vi "VSS_GoTo_Circ.vi"(6 "Npoint":i32, 9 "y 3":dbl=0.5, 10 "SetPoint":dbl[](array[numeric])=[100.0, 100.0, 0.0], 11 "Position":dbl[](array[numeric])=[208.6539306640625, -200.4281768798828, 3.141592653589793]) -> (3 "Output Vel":dbl[](array[numeric])=[0.0, 0.0, 0.8321627905647668])   [LabVIEW 2018]
uses:
  <vilib>/Analysis/_algsub.llb/Real Vector Norm.vi
  <vilib>/Analysis/coordinate.llb/Wrap Angle (scalar).vi
  <vilib>/Analysis/NI_AAL_Angle.lvlib
  <vilib>/Analysis/NI_AALPro.lvlib
panel:
  in  "Beta":dbl=0.17
  in  "Dmin":dbl=250.0
  in  "fc angular":dbl=80.0
  out "Angular":dbl(graph)=0.8321627905647668
  out "Tangent":dbl(graph)
  in  "fc tangent":dbl=0.85
  out "NaN":bool
  in  "y 2":dbl=20.0 format="%#_13g"
  in  "y":dbl=0.6 format="%#_13g"
  in  "Limits tangent":cluster{"output high":dbl, "output low":dbl}={"output high"=1.2, "output low"=-1.2}
  in  "PID gains tangent":T1={"proportional gain (Kc)"=0.0044, "integral time (Ti, min)"=0.0, "derivative time (Td, min)"=-0.085}
  in  "Limits ang":cluster{"output high":dbl, "output low":dbl}={"output high"=1.0, "output low"=-1.0}
  in  "PID gains ang":T1={"proportional gain (Kc)"=0.5, "integral time (Ti, min)"=0.0, "derivative time (Td, min)"=-0.08}
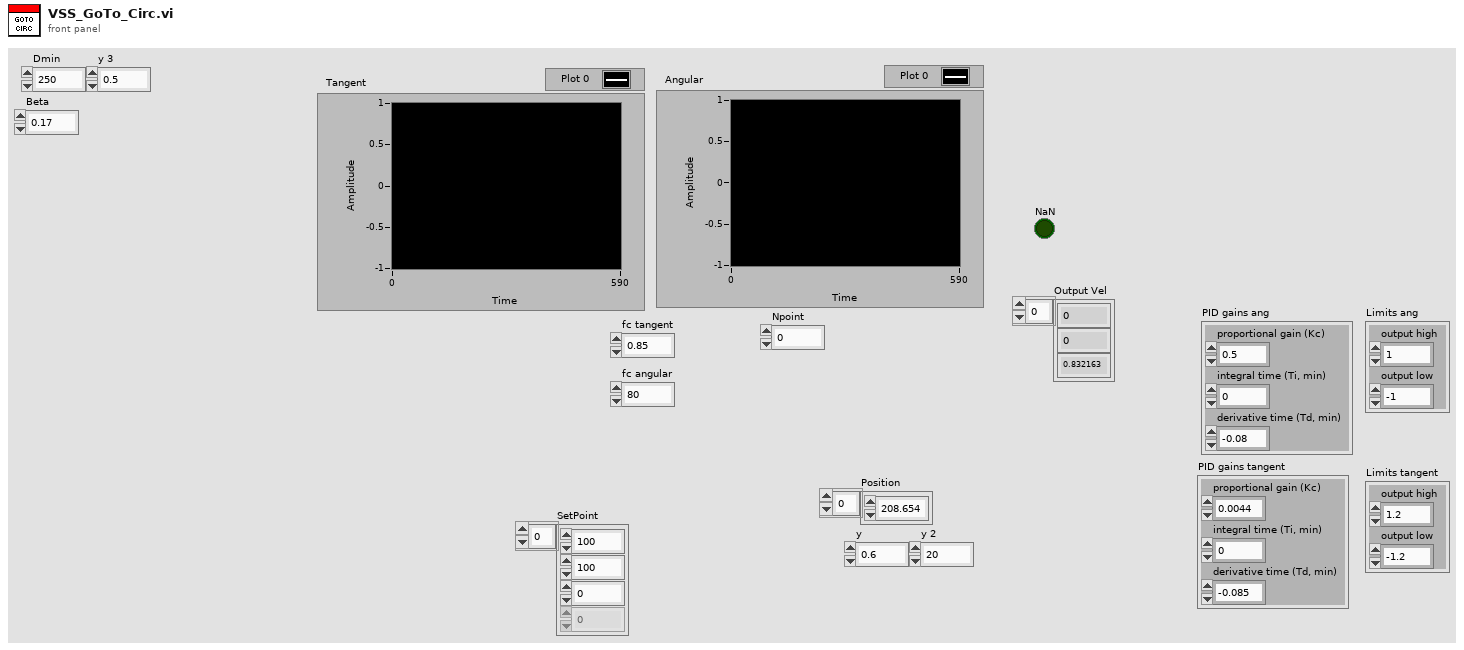
[diagram p1: front panel]
types:
  T1 = cluster{"proportional gain (Kc)":dbl, "integral time (Ti, min)":dbl, "derivative time (Td, min)":dbl}
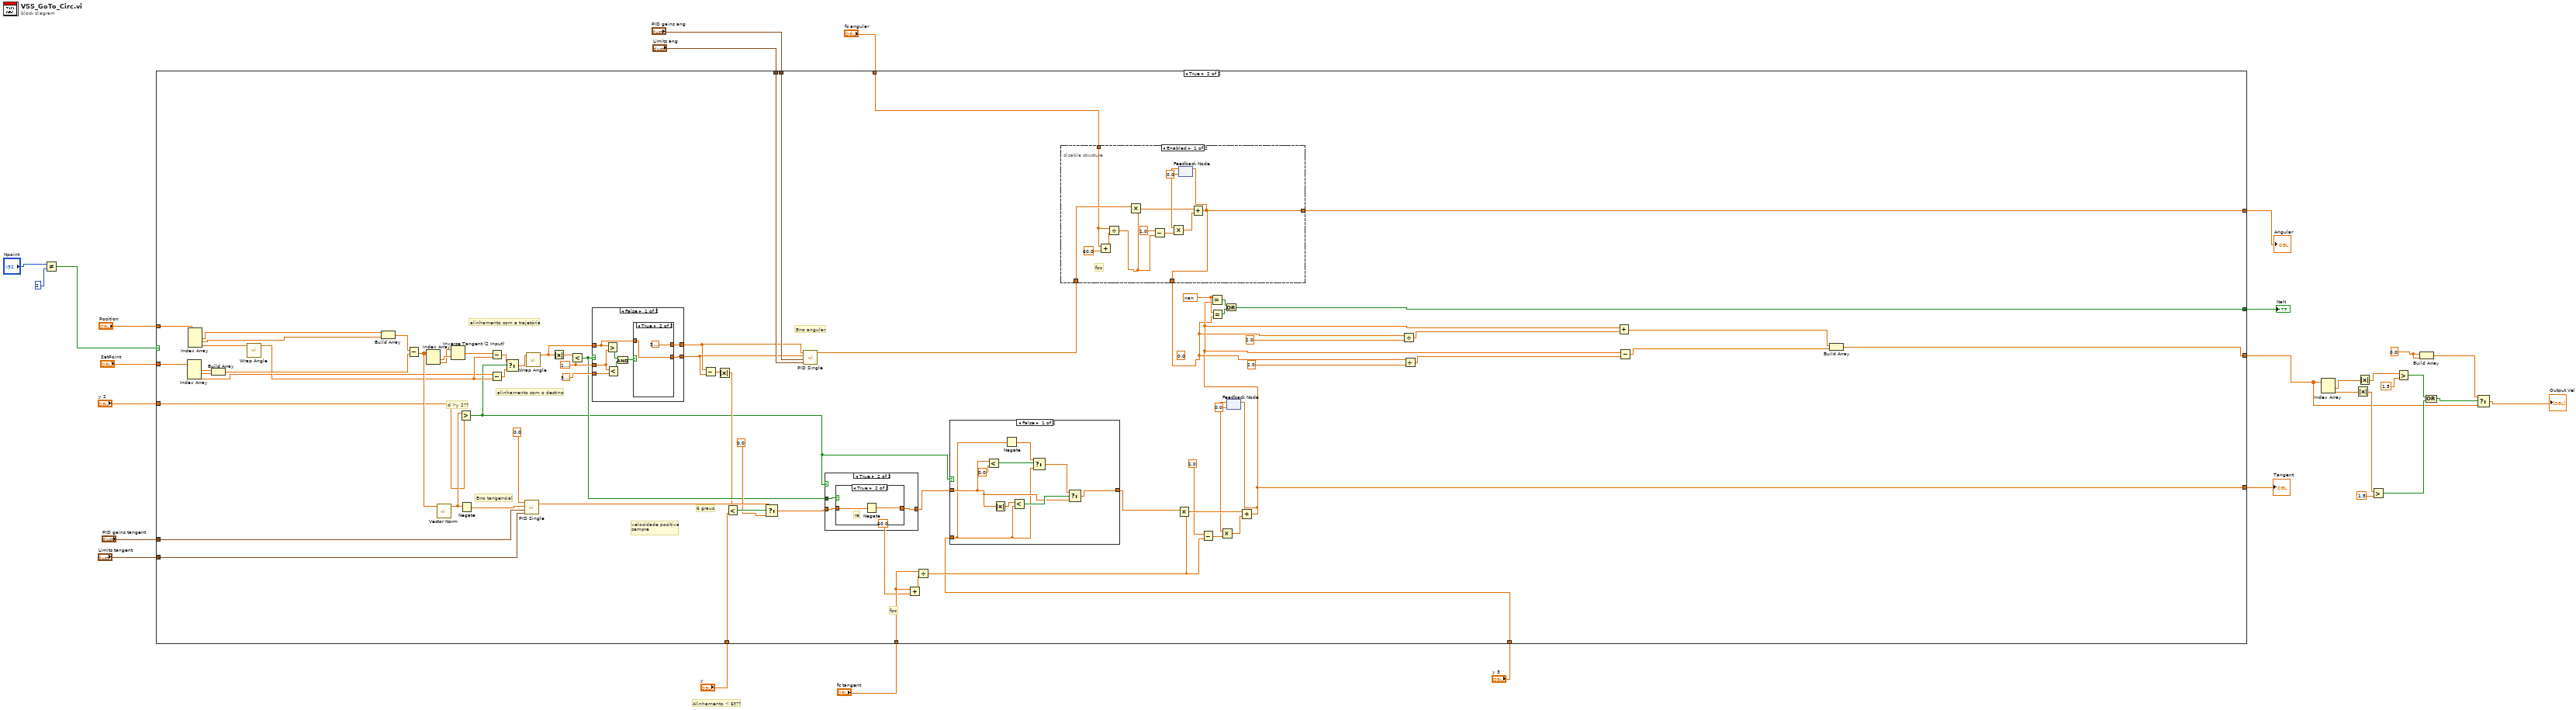
[diagram p0: block diagram]
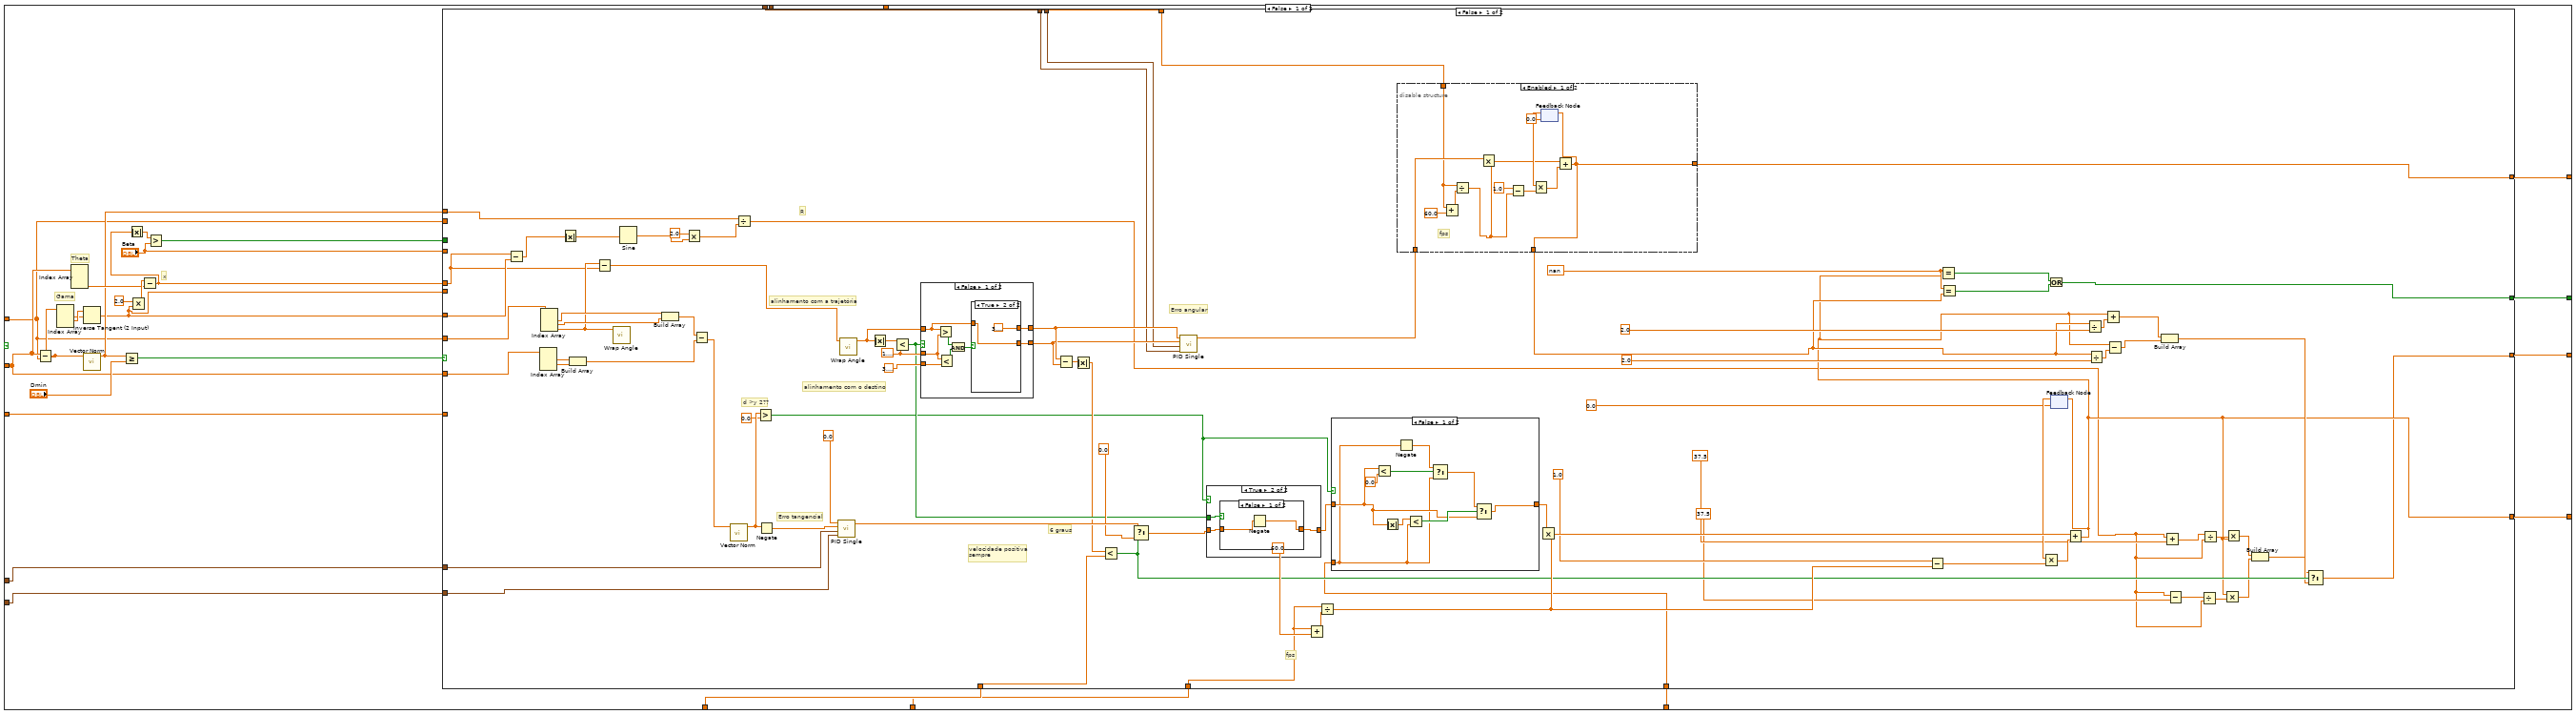
[diagram p2: hidden frame]
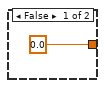
[diagram p5: hidden frame]
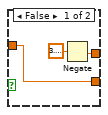
[diagram p7: hidden frame]
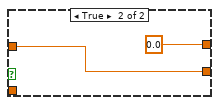
[diagram p8: hidden frame]
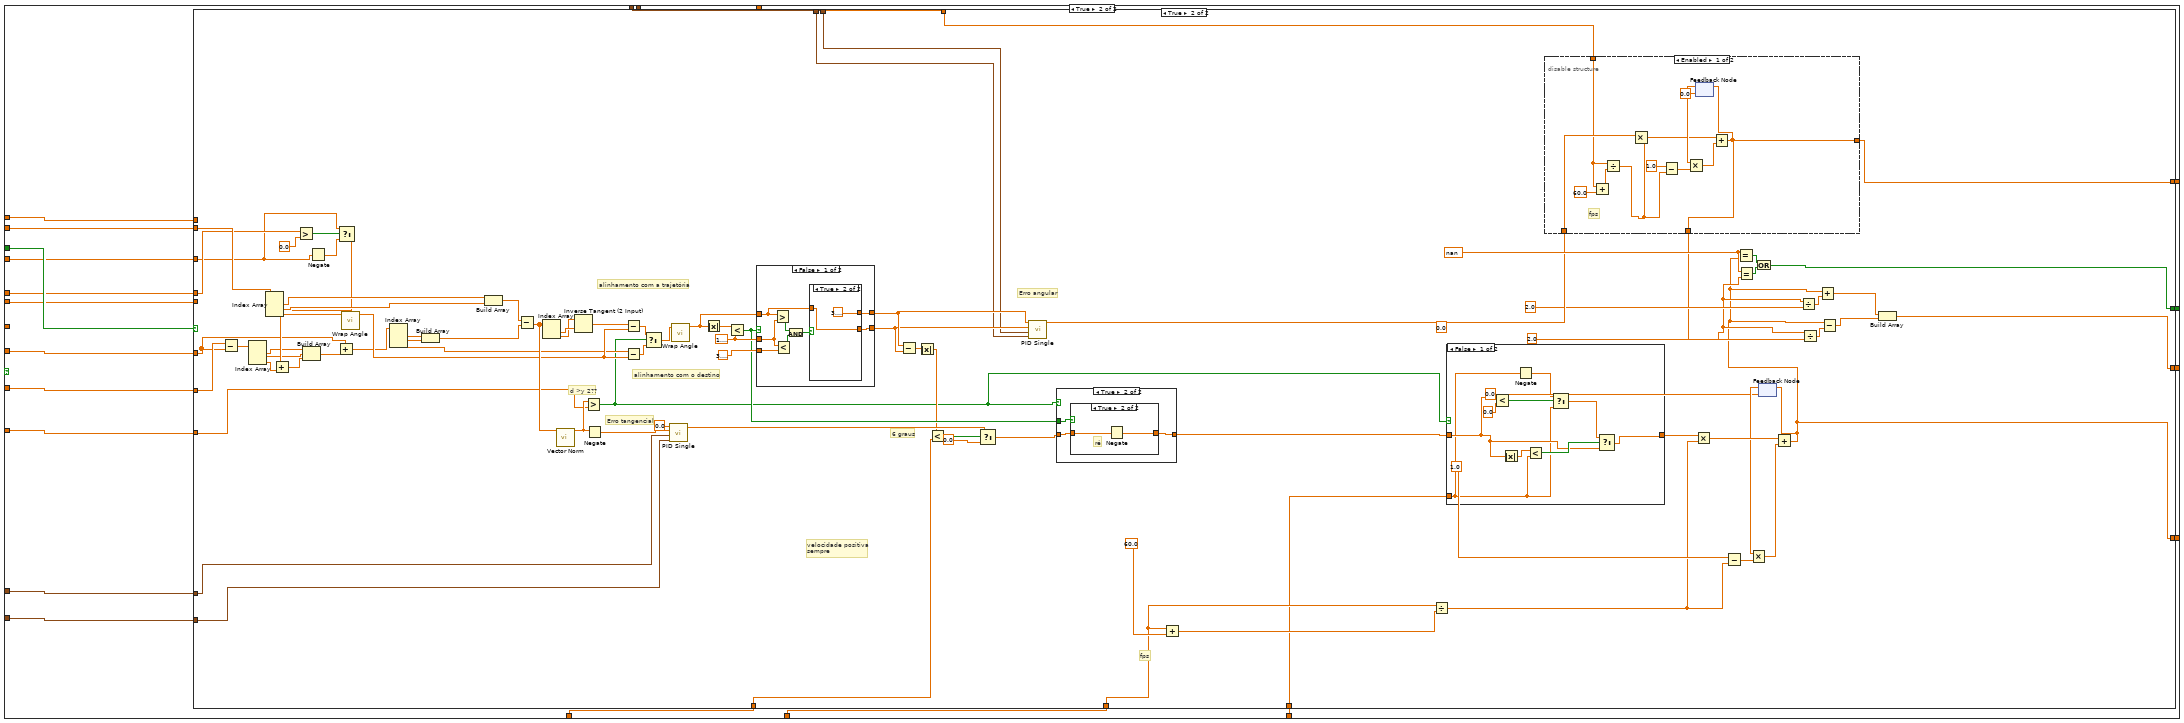
[diagram p9: hidden frame]
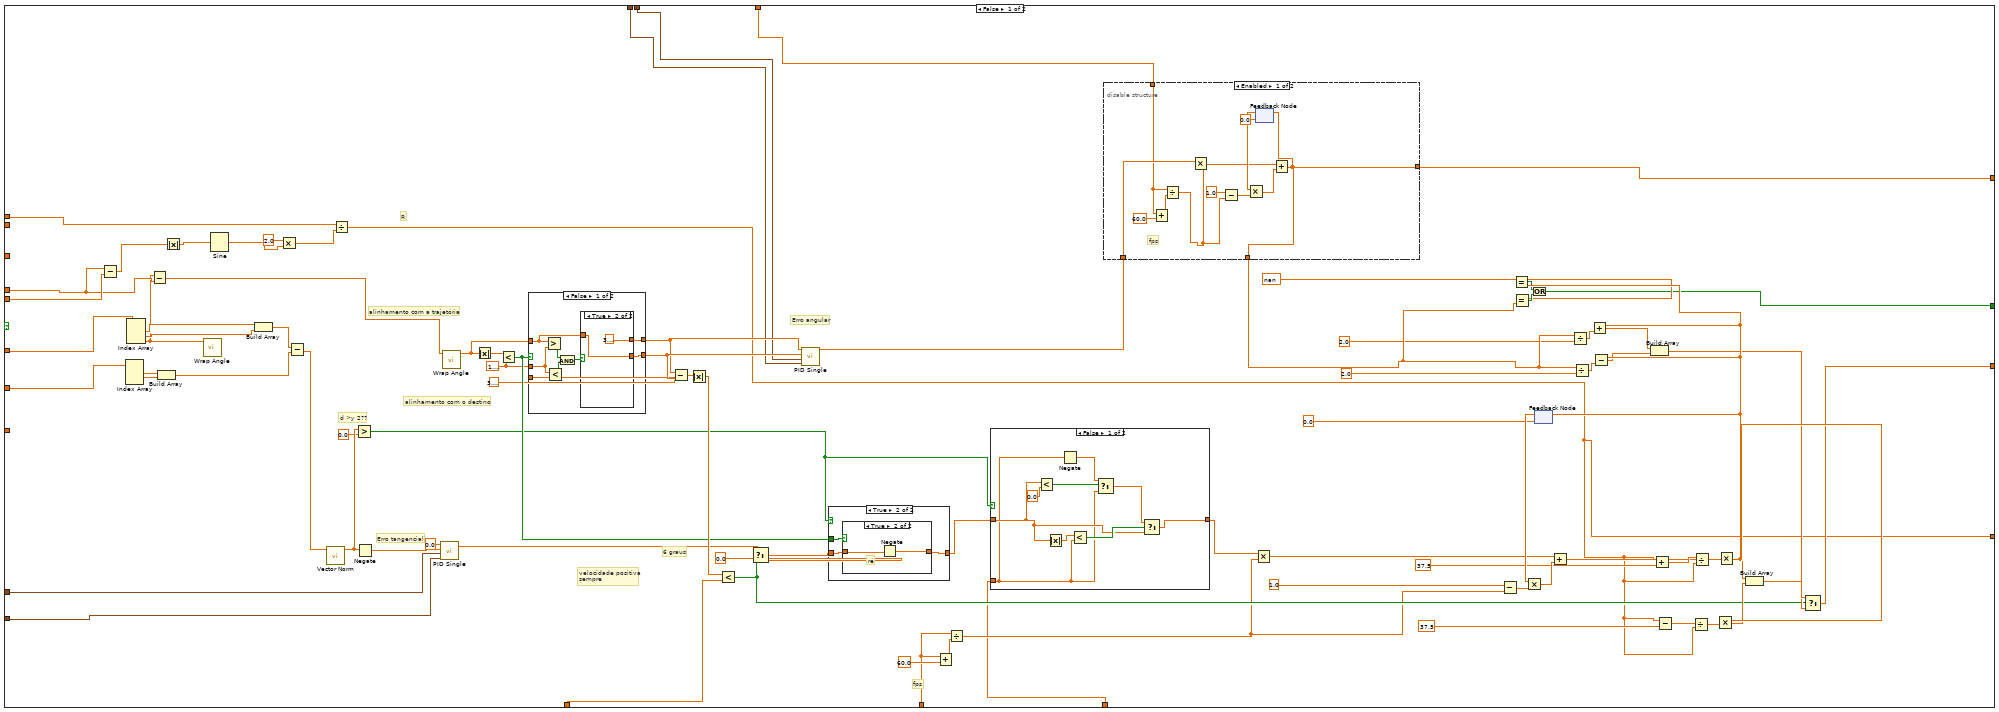
[diagram p10: hidden frame]
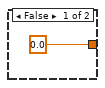
[diagram p13: hidden frame]
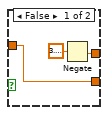
[diagram p15: hidden frame]
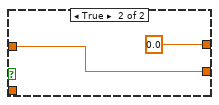
[diagram p16: hidden frame]
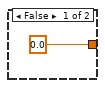
[diagram p19: hidden frame]
diagram:
  w3 = 0.0 ("element")
  # "Alinhamento < 6º??"
  n1 = Not Equal?(x="Npoint", y=2) -> (x != y?=w15:bool)
  n2 = case shown="True" w15 {
    tunnel: "Position" -> [w36 w533]
    tunnel: "PID gains tangent" -> [w50 w528]
    tunnel: "Limits tangent" -> [w51 w527]
    tunnel: "y" -> [w53 w526]
    tunnel: "SetPoint" -> [w48 w520]
    tunnel: "PID gains ang" -> [w46 w516]
    tunnel: "Limits ang" -> [w47 w515]
    tunnel: "y 2" -> [w49 w495]
    tunnel: [w43 w490] -> w22
    tunnel: "fc tangent" -> [w52 w482]
    tunnel: [w41 w470] -> w20
    tunnel: [w42 w468] -> w4
    tunnel: [w44 w478] -> w19
    tunnel: "fc angular" -> [w45 w477]
    tunnel: "y 3" -> [w31 w464]
    frame False {
      # "x"
      # "Theta"
      # "Gama"
      n3 = Subtract(x=w48, y=w36) -> (x-y=w57:dbl[])
      n4 = Index Array(array=w57) -> (element #1=w33:dbl, element #2=w34:dbl)  [unwired: 3 in, 1 out]
      n5 = Index Array(array=w48) -> (element #3=w54:dbl)  [unwired: 3 in, 2 out]
      n6 = Inverse Tangent (2 Input)(1:w33, 2:w34) -> (0:w32:dbl)
      n7 = call-poly <vilib>:"Vector Norm.vi"("Input Vector"=w57) -> ("norm"=w40:dbl)  [unwired: 9 in, 1 out]
      n8 = Greater Or Equal?(x=w40, y="Dmin") -> (x >= y?=w58:bool)
      n9 = Multiply(x=2.0, y=w32) -> (x*y=w55:dbl)
      n10 = Subtract(x=w55, y=w54) -> (x-y=w38:dbl)
      n11 = Absolute Value(x=w38) -> (abs(x)=w37:dbl)
      n12 = Greater?(x=w37, y="Beta") -> (0:w39:bool)
      n13 = case shown="False" w58 {
        tunnel: w38 -> [w64 w205]
        tunnel: w53 -> [w106 w199]
        tunnel: w52 -> [w105 w198]
        tunnel: w51 -> [w104 w200]
        tunnel: w50 -> [w103 w201]
        tunnel: w49 -> [_ w202]
        tunnel: w36 -> [w102 w204]
        tunnel: w48 -> [w101 w203]
        tunnel: w47 -> [w100 w196]
        tunnel: w46 -> [w99 w197]
        tunnel: w45 -> [w98 w189]
        tunnel: [w97 w190] -> w44
        tunnel: [w96 w195] -> w43
        tunnel: [w71 w194] -> w42
        tunnel: [w75 w193] -> w41
        tunnel: w40 -> [w92 w206]
        tunnel: w39 -> [_ w207]
        tunnel: w36 -> [_ w192]
        tunnel: "Beta" -> [_ w191]
        tunnel: w32 -> [w69 _]
        tunnel: w32 -> [_ w188]
        tunnel: w31 -> [w60 w187]
        frame False {
          w119 = nan
          w131 = 1.5707963267948966
          # "R"
          # "d >y 2??"
          # "fps"
          # "alinhamento com o destino"
          # "alinhamento com a trajetória"
          # "velocidade positiva\nsempre"
          # "Erro tangencial"
          # "Erro angular"
          # "6 graus"
          n14 = Subtract(x=w64, y=w69) -> (x-y=w66:dbl)
          n15 = Index Array(array=w101) -> (element #1=w135:dbl, element #2=w134:dbl)  [unwired: 3 in, 1 out]
          n16 = Index Array(array=w102) -> (element #1=w137:dbl, element #2=w136:dbl, element #3=w65:dbl)  [unwired: 3 in]
          n17 = Absolute Value(x=w66) -> (abs(x)=w67:dbl)
          n18 = Build Array(w135, w134) -> (w133:dbl[])
          n19 = Subtract(x=w65, y=w64) -> (x-y=w68:dbl)
          n20 = call-poly <vilib>:"Wrap Angle.vi"("angle in"=w65) -> ()  [unwired: 9 in, 2 out]
          n21 = Sine(x=w67) -> (sin(x)=w94:dbl)
          n22 = Build Array(w137, w136) -> (w141:dbl[])
          n23 = Multiply(x=2.0, y=w94) -> (x*y=w93:dbl)
          n24 = Subtract(x=w141, y=w133) -> (x-y=w122:dbl[])
          n25 = call-poly <vilib>:"Vector Norm.vi"("Input Vector"=w122) -> ("norm"=w121:dbl)  [unwired: 9 in, 1 out]
          n26 = Divide(x=w92, y=w93) -> (x/y=w72:dbl)
          n27 = Greater?(x=w121, y=0.0) -> (0:w61:bool)
          n28 = Negate(x=w121) -> (-x=w126:dbl)
          n29 = call "PID Single.vi"("Limits"=w104, "PID gains in"=w103, "Variable"=w126, "Setpoint"=0.0) -> ("Out"=w139:dbl)  [unwired: 7 in]
          n30 = call-poly <vilib>:"Wrap Angle.vi"("angle in"=w68) -> ("angle out"=w129:dbl)  [unwired: 9 in, 1 out]
          n31 = Absolute Value(x=w129) -> (abs(x)=w132:dbl)
          n32 = Less?(x=w132, y=w131) -> (x < y?=w127:bool)
          n33 = case shown="False" w127 {
            tunnel: w129 -> [w172 w186]
            tunnel: [w173 w186] -> w124
            tunnel: w131 -> [w179 _]
            tunnel: 3.141592653589793 -> [w178 _]
            tunnel: [w174 0.0 ("Variable")] -> w125
            frame False {
              n34 = Greater?(x=w172, y=w179) -> (0:w176:bool)
              n35 = Less?(x=w179, y=w178) -> (x < y?=w177:bool)
              n36 = And(x=w176, y=w177) -> (x .and. y?=w175:bool)
              n37 = case shown="True" w175 {
                tunnel: [w182 3.141592653589793] -> w174
                tunnel: [w180 w183] -> w173
                tunnel: w172 -> [w180 w183]
                frame False {
                  n38 = Negate(x=3.141592653589793) -> (-x=w182:dbl)
                }
                frame True {
                }
              }
            }
            frame True {
            }
          }
          n39 = Subtract(x=w125, y=w124) -> (x-y=w123:dbl)
          n40 = Absolute Value(x=w123) -> (abs(x)=w120:dbl)
          n41 = Less?(x=w120, y=w106) -> (x < y?=w87:bool)
          n42 = Select(t=w139, s=w87, f=0.0) -> (s? t:f=w128:dbl)
          n43 = call "PID Single.vi"("Limits"=w100, "PID gains in"=w99, "Variable"=w124, "Setpoint"=w125) -> ("Out"=w107:dbl)  [unwired: 7 in]
          n44 = case shown="True" w61 {
            tunnel: w128 -> [_ w168]
            tunnel: w127 -> [_ w167]
            tunnel: [0.0 ("f") w166] -> w62
            frame False {
            }
            frame True {
              n45 = case shown="False" w167 {
                tunnel: w168 -> [w170 w171]
                tunnel: [w169 w171] -> w166
                frame False {
                  n46 = Negate(x=w170) -> (-x=w169:dbl)
                }
                frame True {
                  # "ré"
                }
              }
            }
          }
          n47 = Add(x=w105, y=60.0) -> (x+y=w108:dbl)
          n48 = Divide(x=w105, y=w108) -> (x/y=w110:dbl)
          n49 = case shown="False" w61 {
            tunnel: w62 -> [w144 w151]
            tunnel: w60 -> [w143 _]
            tunnel: [w142 w151] -> w63
            frame False {
              n50 = Less?(x=w144, y=0.0) -> (x < y?=w147:bool)
              n51 = Absolute Value(x=w144) -> (abs(x)=w150:dbl)
              n52 = Negate(x=w143) -> (-x=w146:dbl)
              n53 = Less?(x=w150, y=w143) -> (x < y?=w149:bool)
              n54 = Select(t=w146, s=w147, f=w143) -> (s? t:f=w145:dbl)
              n55 = Select(t=w145, s=w149, f=w144) -> (s? t:f=w142:dbl)
            }
            frame True {
            }
          }
          n56 = disable-structure shown="Enabled" {
            disable-tunnel: [w153 w164] -> w86
            disable-tunnel: w107 -> [w154 w164]
            disable-tunnel: [w153 _] -> w97
            disable-tunnel: w98 -> [w152 _]
            frame Enabled {
              # "fps"
              n57 = Add(x=w152, y=60.0) -> (x+y=w157:dbl)
              n58 = Divide(x=w152, y=w157) -> (x/y=w155:dbl)
              n59 = Multiply(x=w154, y=w155) -> (x*y=w158:dbl)
              n60 = Subtract(x=1.0, y=w155) -> (x-y=w160:dbl)
              n61 = feedback #1(0.0) -> (w161:dbl)
              n62 = Multiply(x=w161, y=w160) -> (x*y=w162:dbl)
              n63 = Add(x=w158, y=w162) -> (x+y=w153:dbl)
              n64 = feedback-in #1(w153) -> ()
            }
            frame Disabled {
            }
          }
          n65 = Multiply(x=w63, y=w110) -> (x*y=w116:dbl)
          n66 = Subtract(x=1.0, y=w110) -> (x-y=w114:dbl)
          n67 = Equal?(x=w119, y=w86) -> (x = y?=w118:bool)
          n68 = feedback #2(0.0) -> (w113:dbl)
          n69 = Multiply(x=w113, y=w114) -> (x*y=w112:dbl)
          n70 = Add(x=w116, y=w112) -> (x+y=w75:dbl)
          n71 = Equal?(x=w119, y=w75) -> (x = y?=w117:bool)
          n72 = Or(x=w117, y=w118) -> (x .or. y?=w96:bool)
          n73 = feedback-in #2(w75) -> ()
          n74 = Divide(x=w86, y=2.0) -> (x/y=w88:dbl)
          n75 = Divide(x=w86, y=2.0) -> (x/y=w91:dbl)
          n76 = Add(x=w75, y=w88) -> (x+y=w85:dbl)
          n77 = Subtract(x=w75, y=w91) -> (x-y=w84:dbl)
          n78 = Build Array(w85, w84) -> (w83:dbl[])
          n79 = Add(x=w72, y=37.5) -> (x+y=w73:dbl)
          n80 = Subtract(x=w72, y=37.5) -> (x-y=w74:dbl)
          n81 = Divide(x=w74, y=w72) -> (x/y=w80:dbl)
          n82 = Divide(x=w73, y=w72) -> (x/y=w76:dbl)
          n83 = Multiply(x=w75, y=w80) -> (x*y=w79:dbl)
          n84 = Multiply(x=w76, y=w75) -> (x*y=w78:dbl)
          n85 = Build Array(w78, w79) -> (w77:dbl[])
          n86 = Select(t=w77, s=w87, f=w83) -> (s? t:f=w71:dbl[])
        }
        frame True {
          n87 = case shown="True" w207 {
            tunnel: w206 -> [w232 _]
            tunnel: w205 -> [w213 w361]
            tunnel: w204 -> [w231 w350]
            tunnel: w203 -> [w230 w357]
            tunnel: w202 -> [_ w364]
            tunnel: w201 -> [w229 w365]
            tunnel: w200 -> [w228 w366]
            tunnel: w199 -> [w227 w347]
            tunnel: w198 -> [w226 w346]
            tunnel: w197 -> [w224 w340]
            tunnel: w196 -> [w223 w341]
            tunnel: [w222 w345] -> w195
            tunnel: [w221 w343] -> w194
            tunnel: [w220 w342] -> w193
            tunnel: w192 -> [_ w363]
            tunnel: w191 -> [_ w359]
            tunnel: [w219 w344] -> w190
            tunnel: w189 -> [w225 w339]
            tunnel: w188 -> [w217 _]
            tunnel: w187 -> [w209 w335]
            frame False {
              w241 = nan
              w245 = 1.5707963267948966
              # "R"
              # "d >y 2??"
              # "fps"
              # "alinhamento com o destino"
              # "alinhamento com a trajetória"
              # "velocidade positiva\nsempre"
              # "Erro tangencial"
              # "Erro angular"
              # "6 graus"
              n88 = Subtract(x=w213, y=w217) -> (x-y=w215:dbl)
              n89 = Index Array(array=w230) -> (element #1=w250:dbl, element #2=w251:dbl)  [unwired: 3 in, 1 out]
              n90 = Index Array(array=w231) -> (element #1=w248:dbl, element #2=w249:dbl, element #3=w212:dbl)  [unwired: 3 in]
              n91 = Subtract(x=w212, y=w213) -> (x-y=w216:dbl)
              n92 = Build Array(w250, w251) -> (w252:dbl[])
              n93 = Absolute Value(x=w215) -> (abs(x)=w214:dbl)
              n94 = call-poly <vilib>:"Wrap Angle.vi"("angle in"=w212) -> ()  [unwired: 9 in, 2 out]
              n95 = Sine(x=w214) -> (sin(x)=w273:dbl)
              n96 = Build Array(w248, w249) -> (w246:dbl[])
              n97 = Multiply(x=2.0, y=w273) -> (x*y=w274:dbl)
              n98 = Subtract(x=w246, y=w252) -> (x-y=w261:dbl[])
              n99 = call-poly <vilib>:"Vector Norm.vi"("Input Vector"=w261) -> ("norm"=w262:dbl)  [unwired: 9 in, 1 out]
              n100 = Divide(x=w232, y=w274) -> (x/y=w220:dbl)
              n101 = Greater?(x=w262, y=0.0) -> (0:w211:bool)
              n102 = Negate(x=w262) -> (-x=w257:dbl)
              n103 = call "PID Single.vi"("Limits"=w228, "PID gains in"=w229, "Variable"=w257, "Setpoint"=0.0) -> ("Out"=w247:dbl)  [unwired: 7 in]
              n104 = call-poly <vilib>:"Wrap Angle.vi"("angle in"=w216) -> ("angle out"=w254:dbl)  [unwired: 9 in, 1 out]
              n105 = Absolute Value(x=w254) -> (abs(x)=w253:dbl)
              n106 = Less?(x=w253, y=w245) -> (x < y?=w256:bool)
              n107 = case shown="False" w256 {
                tunnel: w254 -> [w320 w334]
                tunnel: [w321 w334] -> w259
                tunnel: w245 -> [w327 _]
                tunnel: 3.141592653589793 -> [w326 _]
                tunnel: [w322 0.0 ("Variable")] -> w258
                frame False {
                  n108 = Greater?(x=w320, y=w327) -> (0:w324:bool)
                  n109 = Less?(x=w327, y=w326) -> (x < y?=w325:bool)
                  n110 = And(x=w324, y=w325) -> (x .and. y?=w323:bool)
                  n111 = case shown="True" w323 {
                    tunnel: [w330 3.141592653589793] -> w322
                    tunnel: [w328 w331] -> w321
                    tunnel: w320 -> [w328 w331]
                    frame False {
                      n112 = Negate(x=3.141592653589793) -> (-x=w330:dbl)
                    }
                    frame True {
                    }
                  }
                }
                frame True {
                }
              }
              n113 = Subtract(x=w258, y=w259) -> (x-y=w260:dbl)
              n114 = Absolute Value(x=w260) -> (abs(x)=w263:dbl)
              n115 = Less?(x=w263, y=w227) -> (x < y?=w277:bool)
              n116 = Select(t=w247, s=w277, f=0.0) -> (s? t:f=w255:dbl)
              n117 = call "PID Single.vi"("Limits"=w223, "PID gains in"=w224, "Variable"=w259, "Setpoint"=w258) -> ("Out"=w272:dbl)  [unwired: 7 in]
              n118 = case shown="True" w211 {
                tunnel: w255 -> [_ w316]
                tunnel: w256 -> [_ w315]
                tunnel: [0.0 ("f") w314] -> w208
                frame False {
                }
                frame True {
                  n119 = case shown="True" w315 {
                    tunnel: w316 -> [w317 w319]
                    tunnel: [w317 w318] -> w314
                    frame False {
                    }
                    frame True {
                      # "ré"
                      n120 = Negate(x=w319) -> (-x=w318:dbl)
                    }
                  }
                }
              }
              n121 = Add(x=w226, y=60.0) -> (x+y=w271:dbl)
              n122 = Divide(x=w226, y=w271) -> (x/y=w270:dbl)
              n123 = case shown="False" w211 {
                tunnel: w208 -> [w292 w299]
                tunnel: w209 -> [w291 _]
                tunnel: [w290 w299] -> w210
                frame False {
                  n124 = Less?(x=w292, y=0.0) -> (x < y?=w295:bool)
                  n125 = Absolute Value(x=w292) -> (abs(x)=w298:dbl)
                  n126 = Negate(x=w291) -> (-x=w294:dbl)
                  n127 = Less?(x=w298, y=w291) -> (x < y?=w297:bool)
                  n128 = Select(t=w294, s=w295, f=w291) -> (s? t:f=w293:dbl)
                  n129 = Select(t=w293, s=w297, f=w292) -> (s? t:f=w290:dbl)
                }
                frame True {
                }
              }
              n130 = disable-structure shown="Enabled" {
                disable-tunnel: [w301 w312] -> w278
                disable-tunnel: w272 -> [w302 w312]
                disable-tunnel: [w301 _] -> w219
                disable-tunnel: w225 -> [w300 _]
                frame Enabled {
                  # "fps"
                  n131 = Add(x=w300, y=60.0) -> (x+y=w305:dbl)
                  n132 = Divide(x=w300, y=w305) -> (x/y=w303:dbl)
                  n133 = Multiply(x=w302, y=w303) -> (x*y=w306:dbl)
                  n134 = Subtract(x=1.0, y=w303) -> (x-y=w308:dbl)
                  n135 = feedback #3(0.0) -> (w309:dbl)
                  n136 = Multiply(x=w309, y=w308) -> (x*y=w310:dbl)
                  n137 = Add(x=w306, y=w310) -> (x+y=w301:dbl)
                  n138 = feedback-in #3(w301) -> ()
                }
                frame Disabled {
                }
              }
              n139 = Multiply(x=w210, y=w270) -> (x*y=w266:dbl)
              n140 = Subtract(x=1.0, y=w270) -> (x-y=w267:dbl)
              n141 = Equal?(x=w241, y=w278) -> (x = y?=w264:bool)
              n142 = feedback #4(0.0) -> (w268:dbl)
              n143 = Multiply(x=w268, y=w267) -> (x*y=w269:dbl)
              n144 = Add(x=w266, y=w269) -> (x+y=w287:dbl)
              n145 = Equal?(x=w241, y=w287) -> (x = y?=w265:bool)
              n146 = Or(x=w265, y=w264) -> (x .or. y?=w222:bool)
              n147 = feedback-in #4(w287) -> ()
              n148 = Divide(x=w278, y=2.0) -> (x/y=w276:dbl)
              n149 = Divide(x=w278, y=2.0) -> (x/y=w275:dbl)
              n150 = Add(x=w287, y=w276) -> (x+y=w279:dbl)
              n151 = Subtract(x=w287, y=w275) -> (x-y=w280:dbl)
              n152 = Build Array(w279, w280) -> (w281:dbl[])
              n153 = Add(x=w220, y=37.5) -> (x+y=w289:dbl)
              n154 = Subtract(x=w220, y=37.5) -> (x-y=w288:dbl)
              n155 = Divide(x=w288, y=w220) -> (x/y=w282:dbl)
              n156 = Divide(x=w289, y=w220) -> (x/y=w286:dbl)
              n157 = Multiply(x=w287, y=w282) -> (x*y=w283:dbl)
              n158 = Multiply(x=w286, y=w287) -> (x*y=w284:dbl)
              n159 = Build Array(w284, w283) -> (w285:dbl[])
              n160 = Select(t=w285, s=w277, f=w281) -> (s? t:f=w221:dbl[])
            }
            frame True {
              w386 = nan
              w404 = 1.5707963267948966
              (unwired) 0.0 ("element")
              # "d >y 2??"
              # "fps"
              # "alinhamento com o destino"
              # "alinhamento com a trajetória"
              # "velocidade positiva\nsempre"
              # "Erro tangencial"
              # "Erro angular"
              # "6 graus"
              n161 = Subtract(x=w357, y=w350) -> (x-y=w356:dbl[])
              n162 = Index Array(array=w356) -> (element #1=w353:dbl, element #2=w352:dbl, element #3=w354:dbl)  [unwired: 3 in]
              n163 = Index Array(array=w363) -> (element #1=w411:dbl, element #2=w410:dbl, element #3=w406:dbl)  [unwired: 3 in]
              n164 = Greater?(x=w361, y=0.0) -> (0:w360:bool)
              n165 = Negate(x=w359) -> (-x=w358:dbl)
              n166 = Select(t=w359, s=w360, f=w358) -> (s? t:f=w355:dbl)
              n167 = Add(x=w355, y=w354) -> (x+y=w351:dbl)
              n168 = Build Array(w353, w352, w351) -> (w349:dbl[])
              n169 = Add(x=w350, y=w349) -> (x+y=w348:dbl[])
              n170 = call-poly <vilib>:"Wrap Angle.vi"("angle in"=w406) -> ("angle out"=w393:dbl)  [unwired: 9 in, 1 out]
              n171 = Index Array(array=w348) -> (element #1=w409:dbl, element #2=w408:dbl, element #3=w392:dbl)  [unwired: 3 in]
              n172 = Build Array(w409, w408) -> (w407:dbl[])
              n173 = Build Array(w411, w410) -> (w418:dbl[])
              n174 = Subtract(x=w418, y=w407) -> (x-y=w395:dbl[])
              n175 = Index Array(array=w395) -> (element #1=w417:dbl, element #2=w416:dbl)  [unwired: 2 in]
              n176 = call-poly <vilib>:"Vector Norm.vi"("Input Vector"=w395) -> ("norm"=w388:dbl)  [unwired: 9 in, 1 out]
              n177 = Inverse Tangent (2 Input)(1:w417, 2:w416) -> (0:w394:dbl)
              n178 = Greater?(x=w388, y=w364) -> (0:w336:bool)
              n179 = Negate(x=w388) -> (-x=w399:dbl)
              n180 = Subtract(x=w394, y=w393) -> (x-y=w390:dbl)
              n181 = Subtract(x=w392, y=w393) -> (x-y=w389:dbl)
              n182 = Select(t=w390, s=w336, f=w389) -> (s? t:f=w391:dbl)
              n183 = call "PID Single.vi"("Limits"=w366, "PID gains in"=w365, "Variable"=w399, "Setpoint"=0.0) -> ("Out"=w413:dbl)  [unwired: 7 in]
              n184 = call-poly <vilib>:"Wrap Angle.vi"("angle in"=w391) -> ("angle out"=w402:dbl)  [unwired: 9 in, 1 out]
              n185 = Absolute Value(x=w402) -> (abs(x)=w405:dbl)
              n186 = Less?(x=w405, y=w404) -> (x < y?=w400:bool)
              n187 = case shown="False" w400 {
                tunnel: w402 -> [w449 w463]
                tunnel: [w450 w463] -> w397
                tunnel: w404 -> [w456 _]
                tunnel: 3.141592653589793 -> [w455 _]
                tunnel: [w451 0.0 ("Variable")] -> w398
                frame False {
                  n188 = Greater?(x=w449, y=w456) -> (0:w453:bool)
                  n189 = Less?(x=w456, y=w455) -> (x < y?=w454:bool)
                  n190 = And(x=w453, y=w454) -> (x .and. y?=w452:bool)
                  n191 = case shown="True" w452 {
                    tunnel: [w459 3.141592653589793] -> w451
                    tunnel: [w457 w460] -> w450
                    tunnel: w449 -> [w457 w460]
                    frame False {
                      n192 = Negate(x=3.141592653589793) -> (-x=w459:dbl)
                    }
                    frame True {
                    }
                  }
                }
                frame True {
                }
              }
              n193 = Subtract(x=w398, y=w397) -> (x-y=w396:dbl)
              n194 = Absolute Value(x=w396) -> (abs(x)=w387:dbl)
              n195 = Less?(x=w387, y=w347) -> (x < y?=w414:bool)
              n196 = Select(t=w413, s=w414, f=0.0) -> (s? t:f=w401:dbl)
              n197 = call "PID Single.vi"("Limits"=w341, "PID gains in"=w340, "Variable"=w397, "Setpoint"=w398) -> ("Out"=w374:dbl)  [unwired: 7 in]
              n198 = case shown="True" w336 {
                tunnel: w401 -> [_ w445]
                tunnel: w400 -> [_ w444]
                tunnel: [0.0 ("f") w443] -> w338
                frame False {
                }
                frame True {
                  n199 = case shown="True" w444 {
                    tunnel: w445 -> [w446 w448]
                    tunnel: [w446 w447] -> w443
                    frame False {
                    }
                    frame True {
                      # "ré"
                      n200 = Negate(x=w448) -> (-x=w447:dbl)
                    }
                  }
                }
              }
              n201 = Add(x=w346, y=60.0) -> (x+y=w375:dbl)
              n202 = Divide(x=w346, y=w375) -> (x/y=w377:dbl)
              n203 = case shown="False" w336 {
                tunnel: w338 -> [w421 w428]
                tunnel: w335 -> [w420 _]
                tunnel: [w419 w428] -> w337
                frame False {
                  n204 = Less?(x=w421, y=0.0) -> (x < y?=w424:bool)
                  n205 = Absolute Value(x=w421) -> (abs(x)=w427:dbl)
                  n206 = Negate(x=w420) -> (-x=w423:dbl)
                  n207 = Less?(x=w427, y=w420) -> (x < y?=w426:bool)
                  n208 = Select(t=w423, s=w424, f=w420) -> (s? t:f=w422:dbl)
                  n209 = Select(t=w422, s=w426, f=w421) -> (s? t:f=w419:dbl)
                }
                frame True {
                }
              }
              n210 = disable-structure shown="Enabled" {
                disable-tunnel: [w430 w441] -> w367
                disable-tunnel: w374 -> [w431 w441]
                disable-tunnel: [w430 _] -> w344
                disable-tunnel: w339 -> [w429 _]
                frame Enabled {
                  # "fps"
                  n211 = Add(x=w429, y=60.0) -> (x+y=w434:dbl)
                  n212 = Divide(x=w429, y=w434) -> (x/y=w432:dbl)
                  n213 = Multiply(x=w431, y=w432) -> (x*y=w435:dbl)
                  n214 = Subtract(x=1.0, y=w432) -> (x-y=w437:dbl)
                  n215 = feedback #5(0.0) -> (w438:dbl)
                  n216 = Multiply(x=w438, y=w437) -> (x*y=w439:dbl)
                  n217 = Add(x=w435, y=w439) -> (x+y=w430:dbl)
                  n218 = feedback-in #5(w430) -> ()
                }
                frame Disabled {
                }
              }
              n219 = Multiply(x=w337, y=w377) -> (x*y=w383:dbl)
              n220 = Subtract(x=1.0, y=w377) -> (x-y=w381:dbl)
              n221 = Equal?(x=w386, y=w367) -> (x = y?=w385:bool)
              n222 = feedback #6(0.0) -> (w380:dbl)
              n223 = Multiply(x=w380, y=w381) -> (x*y=w379:dbl)
              n224 = Add(x=w383, y=w379) -> (x+y=w342:dbl)
              n225 = Equal?(x=w386, y=w342) -> (x = y?=w384:bool)
              n226 = Or(x=w384, y=w385) -> (x .or. y?=w345:bool)
              n227 = feedback-in #6(w342) -> ()
              n228 = Divide(x=w367, y=2.0) -> (x/y=w370:dbl)
              n229 = Divide(x=w367, y=2.0) -> (x/y=w373:dbl)
              n230 = Add(x=w342, y=w370) -> (x+y=w369:dbl)
              n231 = Subtract(x=w342, y=w373) -> (x-y=w368:dbl)
              n232 = Build Array(w369, w368) -> (w343:dbl[])
            }
          }
        }
      }
    }
    frame True {
      w493 = nan
      w512 = 1.5707963267948966
      (unwired) 0.0 ("element")
      # "d >y 2??"
      # "fps"
      # "alinhamento com o destino"
      # "alinhamento com a trajetória"
      # "velocidade positiva\nsempre"
      # "Erro tangencial"
      # "Erro angular"
      # "6 graus"
      n233 = Index Array(array=w520) -> (element #1=w519:dbl, element #2=w518:dbl, element #3=w500:dbl)  [unwired: 3 in]
      n234 = Index Array(array=w533) -> (element #1=w522:dbl, element #2=w521:dbl, element #3=w514:dbl)  [unwired: 3 in]
      n235 = Build Array(w519, w518) -> (w517:dbl[])
      n236 = call-poly <vilib>:"Wrap Angle.vi"("angle in"=w514) -> ("angle out"=w501:dbl)  [unwired: 9 in, 1 out]
      n237 = Build Array(w522, w521) -> (w532:dbl[])
      n238 = Subtract(x=w532, y=w517) -> (x-y=w503:dbl[])
      n239 = Index Array(array=w503) -> (element #1=w531:dbl, element #2=w530:dbl)  [unwired: 2 in]
      n240 = call-poly <vilib>:"Vector Norm.vi"("Input Vector"=w503) -> ("norm"=w496:dbl)  [unwired: 9 in, 1 out]
      n241 = Inverse Tangent (2 Input)(1:w531, 2:w530) -> (0:w502:dbl)
      n242 = Greater?(x=w496, y=w495) -> (0:w465:bool)
      n243 = Negate(x=w496) -> (-x=w507:dbl)
      n244 = Subtract(x=w502, y=w501) -> (x-y=w498:dbl)
      n245 = Subtract(x=w500, y=w501) -> (x-y=w497:dbl)
      n246 = Select(t=w498, s=w465, f=w497) -> (s? t:f=w499:dbl)
      n247 = call "PID Single.vi"("Limits"=w527, "PID gains in"=w528, "Variable"=w507, "Setpoint"=0.0) -> ("Out"=w524:dbl)  [unwired: 7 in]
      n248 = call-poly <vilib>:"Wrap Angle.vi"("angle in"=w499) -> ("angle out"=w510:dbl)  [unwired: 9 in, 1 out]
      n249 = Absolute Value(x=w510) -> (abs(x)=w513:dbl)
      n250 = Less?(x=w513, y=w512) -> (x < y?=w508:bool)
      n251 = case shown="False" w508 {
        tunnel: w510 -> [w564 w578]
        tunnel: [w565 w578] -> w505
        tunnel: w512 -> [w571 _]
        tunnel: 3.141592653589793 -> [w570 _]
        tunnel: [w566 0.0 ("Variable")] -> w506
        frame False {
          n252 = Greater?(x=w564, y=w571) -> (0:w568:bool)
          n253 = Less?(x=w571, y=w570) -> (x < y?=w569:bool)
          n254 = And(x=w568, y=w569) -> (x .and. y?=w567:bool)
          n255 = case shown="True" w567 {
            tunnel: [w574 3.141592653589793] -> w566
            tunnel: [w572 w575] -> w565
            tunnel: w564 -> [w572 w575]
            frame False {
              n256 = Negate(x=3.141592653589793) -> (-x=w574:dbl)
            }
            frame True {
            }
          }
        }
        frame True {
        }
      }
      n257 = Subtract(x=w506, y=w505) -> (x-y=w504:dbl)
      n258 = Absolute Value(x=w504) -> (abs(x)=w494:dbl)
      n259 = Less?(x=w494, y=w526) -> (x < y?=w525:bool)
      n260 = Select(t=w524, s=w525, f=0.0) -> (s? t:f=w509:dbl)
      n261 = call "PID Single.vi"("Limits"=w515, "PID gains in"=w516, "Variable"=w505, "Setpoint"=w506) -> ("Out"=w479:dbl)  [unwired: 7 in]
      n262 = case shown="True" w465 {
        tunnel: w509 -> [_ w560]
        tunnel: w508 -> [_ w559]
        tunnel: [0.0 ("f") w558] -> w466
        frame False {
        }
        frame True {
          n263 = case shown="True" w559 {
            tunnel: w560 -> [w561 w563]
            tunnel: [w561 w562] -> w558
            frame False {
            }
            frame True {
              # "ré"
              n264 = Negate(x=w563) -> (-x=w562:dbl)
            }
          }
        }
      }
      n265 = Add(x=w482, y=60.0) -> (x+y=w480:dbl)
      n266 = Divide(x=w482, y=w480) -> (x/y=w483:dbl)
      n267 = case shown="False" w465 {
        tunnel: w466 -> [w536 w543]
        tunnel: w464 -> [w535 _]
        tunnel: [w534 w543] -> w467
        frame False {
          n268 = Less?(x=w536, y=0.0) -> (x < y?=w539:bool)
          n269 = Absolute Value(x=w536) -> (abs(x)=w542:dbl)
          n270 = Negate(x=w535) -> (-x=w538:dbl)
          n271 = Less?(x=w542, y=w535) -> (x < y?=w541:bool)
          n272 = Select(t=w538, s=w539, f=w535) -> (s? t:f=w537:dbl)
          n273 = Select(t=w537, s=w541, f=w536) -> (s? t:f=w534:dbl)
        }
        frame True {
        }
      }
      n274 = disable-structure shown="Enabled" {
        disable-tunnel: [w545 w556] -> w469
        disable-tunnel: w479 -> [w546 w556]
        disable-tunnel: [w545 _] -> w478
        disable-tunnel: w477 -> [w544 _]
        frame Enabled {
          # "fps"
          n275 = Add(x=w544, y=60.0) -> (x+y=w549:dbl)
          n276 = Divide(x=w544, y=w549) -> (x/y=w547:dbl)
          n277 = Multiply(x=w546, y=w547) -> (x*y=w550:dbl)
          n278 = Subtract(x=1.0, y=w547) -> (x-y=w552:dbl)
          n279 = feedback #7(0.0) -> (w553:dbl)
          n280 = Multiply(x=w553, y=w552) -> (x*y=w554:dbl)
          n281 = Add(x=w550, y=w554) -> (x+y=w545:dbl)
          n282 = feedback-in #7(w545) -> ()
        }
        frame Disabled {
        }
      }
      n283 = Multiply(x=w467, y=w483) -> (x*y=w489:dbl)
      n284 = Subtract(x=1.0, y=w483) -> (x-y=w487:dbl)
      n285 = Equal?(x=w493, y=w469) -> (x = y?=w492:bool)
      n286 = feedback #8(0.0) -> (w486:dbl)
      n287 = Multiply(x=w486, y=w487) -> (x*y=w485:dbl)
      n288 = Add(x=w489, y=w485) -> (x+y=w470:dbl)
      n289 = Equal?(x=w493, y=w470) -> (x = y?=w491:bool)
      n290 = Or(x=w491, y=w492) -> (x .or. y?=w490:bool)
      n291 = feedback-in #8(w470) -> ()
      n292 = Divide(x=w469, y=2.0) -> (x/y=w473:dbl)
      n293 = Divide(x=w469, y=2.0) -> (x/y=w476:dbl)
      n294 = Add(x=w470, y=w473) -> (x+y=w472:dbl)
      n295 = Subtract(x=w470, y=w476) -> (x-y=w471:dbl)
      n296 = Build Array(w472, w471) -> (w468:dbl[])
    }
  }
  "NaN" <- w22
  "Tangent" <- w20
  "Angular" <- w19
  n297 = Index Array(array=w4) -> (element #1=w13:dbl, element #2=w12:dbl)  [unwired: 2 in]
  n298 = Absolute Value(x=w12) -> (abs(x)=w9:dbl)
  n299 = Absolute Value(x=w13) -> (abs(x)=w10:dbl)
  n300 = Greater?(x=w9, y=1.5) -> (0:w7:bool)
  n301 = Greater?(x=w10, y=1.5) -> (0:w8:bool)
  n302 = Build Array(w3, w3) -> (w5:dbl[])
  n303 = Compound Arithmetic op=OR(w8, w7) -> (w6:bool)
  n304 = Select(t=w5, s=w6, f=w4) -> (s? t:f=→"Output Vel":dbl[])
